vi "set color waveform.vi"(0 "WaveformChart in":refnum<vi>, 5 "size":i32, 7 "#ch":i32) -> ()   [LabVIEW 2019, in "GUI Sensor Lib.lvclass"]
uses:
  GUI Sensor Lib.lvclass
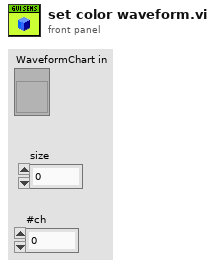
[diagram p1: front panel]
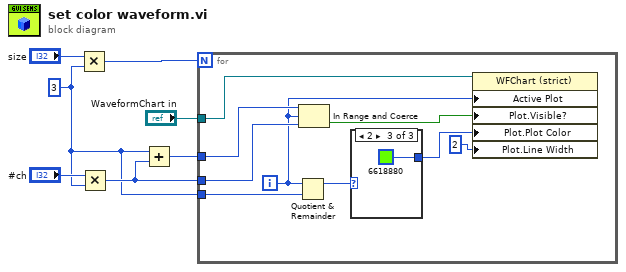
[diagram p0: block diagram]
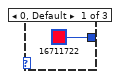
[diagram p2: hidden frame]
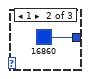
[diagram p3: hidden frame]
diagram:
  w1 = 3 ("x")
  n1 = Multiply(x="size", y=w1) -> (x*y=w4:i32)
  n2 = Multiply(x="#ch", y=w1) -> (x*y=w6:i32)
  n3 = Add(x=w1, y=w6) -> (x+y=w7:i32)
  n4 = for {
    N: w4 -> [_]
    tunnel: "WaveformChart in" -> [w16]
    tunnel: w6 -> [w15]
    tunnel: w7 -> [w14]
    tunnel: w1 -> [w11]
    i -> [w12]
    n5 = Quotient & Remainder(x=w12, y=w11) -> (x-y*floor(x/y)=w10:i32)  [unwired: 1 out]
    n6 = In Range and Coerce(upper limit=w14, x=w12, lower limit=w15) -> (In Range?=w13:bool)  [unwired: 1 out]
    n7 = case shown="2" w10 {
      tunnel: [u32 16711722 u32 16860 u32 6618880] -> w9
      frame 0, Default {
      }
      frame 1 {
      }
      frame 2 {
      }
    }
    n8 = property class="WFChart (strict)"(reference=w16, "Active Plot"=w12, "Plot.Visible?"=w13, "Plot.Plot Color"=w9, "Plot.Line Width"=u8 2) -> ()  [unwired: 1 in, 2 out]
  }
